vi "layout.vi"(0 "reference":refnum<class "RectangularNode.lvclass">, 1 "graph":refnum<class "Graph.lvclass">, 2 "graphics":refnum<class "Graphics.lvclass">, 3 "grid":refnum<class "Grid.lvclass">, 5 "error in (no error)":errorcluster) -> (14 "reference out":refnum<class "RectangularNode.lvclass">, 19 "error out":errorcluster)   [LabVIEW 2014, in "RectangularNode.lvclass"]
doc: "public void layout(Graph g, Graphics2D g2, Grid grid)"
uses:
  <resource>/Framework/Providers/Open_GDS/UML/RectangularNode_class/RectangularNode.lvclass
  <resource>/Framework/Providers/Open_GDS/UML/Graph_class/Graph.lvclass
  <resource>/Framework/Providers/Open_GDS/UML/Graphics_class/Graphics.lvclass
  <resource>/Framework/Providers/Open_GDS/UML/Grid_class/Grid.lvclass
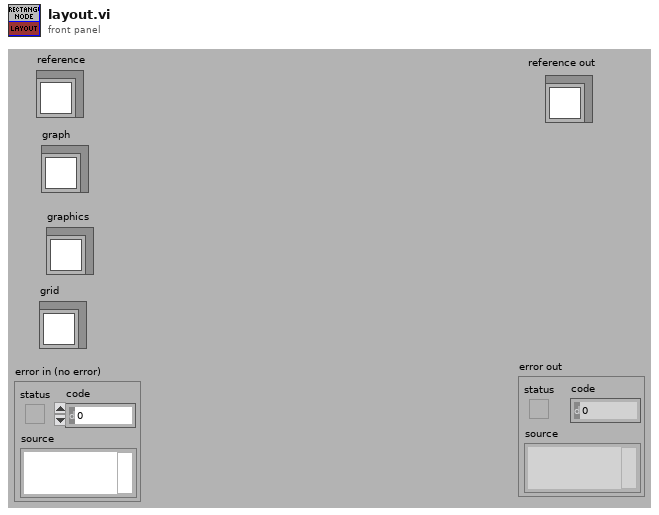
[diagram p1: front panel]
types:
  T1 = typedef "RectangularNode.lvclass/ObjectAttributes.ctl" = cluster{"bounds":T2}
  T2 = typedef "Rectangle Rectangle2D.ctl" = cluster{"x":dbl, "y":dbl, "width":dbl, "height":dbl}
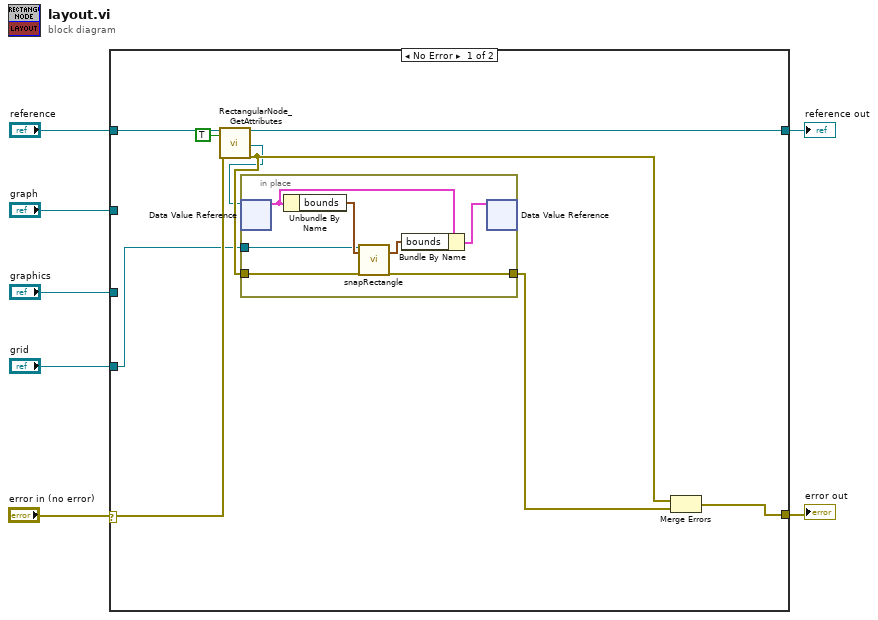
[diagram p0: block diagram]
diagram:
  n1 = case shown="No Error" "error in (no error)" {
    selector: "error in (no error)" -> [w12 w24]
    tunnel: "reference" -> [w16 w25]
    tunnel: [w15 w24] -> w6
    tunnel: [w14 w25] -> w5
    tunnel: "graph" -> [_ _]
    tunnel: "graphics" -> [_ _]
    tunnel: "grid" -> [w9 _]
    frame No Error {
      n2 = call <resource>:"RectangularNode_GetAttributes.vi"("reference in"=w16, "OnlyGetDvrReference(False)"=TRUE, "error in (no error)"=w12) -> ("reference out"=w14:refnum<class "RectangularNode.lvclass">, "DataRef"=w10:refnum<data-value>, "error out"=w13:errorcluster)  [unwired: 13 in, 1 out]
      n3 = in-place {
        in-place-border: w9 -> [w19]
        in-place-border: w13 -> [w18]
        in-place-border: [w17] -> w8
        n4 = in-place-dvr #1(w10) -> (w23:T1)  [unwired: 1 out]
        n5 = Unbundle By Name(w23) -> ("bounds"=w20:T2)
        n6 = call <resource>:"snapRectangle.vi"("reference"=w19, "bounds"=w20, "error in (no error)"=w18) -> ("boundsOut"=w22:T2, "error out"=w17:errorcluster)  [unwired: 15 out]
        n7 = Bundle By Name(cluster=w23, "bounds"=w22) -> (w21:T1)
        n8 = in-place-dvr #1(w21) -> ()  [unwired: 2 out]
      }
      n9 = Merge Errors(w13, w8) -> (w15:errorcluster)
    }
    frame Error {
    }
  }
  "reference out" <- w5
  "error out" <- w6
